vi "Main.vi"() -> ()   [LabVIEW 2012]
uses:
  UIActionQueueElement.ctl
  UIAction.ctl
  MemoryGlobalAction.ctl
  ScanListGlobalAction.ctl
  TriggerConfigurationGlobalAction.ctl
  SlotConfigurationGlobalAction.ctl
  Setup.ctl
  SlotConfiguration.ctl
  BankConfiguration.ctl
  TriggerConfiguration.ctl
  TriggerArmConfiguration.ctl
  driver/Public/Controls/ArmSource.ctl
  TriggerScanConfiguration.ctl
  driver/Public/Controls/ScanSource.ctl
  TriggerChannelConfiguration.ctl
  driver/Public/Controls/TriggerSource.ctl
  HardwareActionQueueElement.ctl
  HardwareAction.ctl
  libs/LV-Utilities/LV-Utilities.lvlib
  driver/Keithley-7001.lvlib
panel:
  in  "Tab Control":enum32{"Page 1"}(tab)
  out "Setup File":path
  in  "CONFIGURE SLOT 1":bool
  in  "CONFIGURE MEMORY":bool
  in  "CONFIGURE SCAN":bool
  in  "CONFIGURE TRIGGER":bool
  in  "Hardware START":bool
  out "Hardware Running?":bool
  in  "RESET":bool
  in  "SAVE":bool
  in  "OPEN":bool
  in  "DONE":bool
  # "RUN"
  # "SETUP"
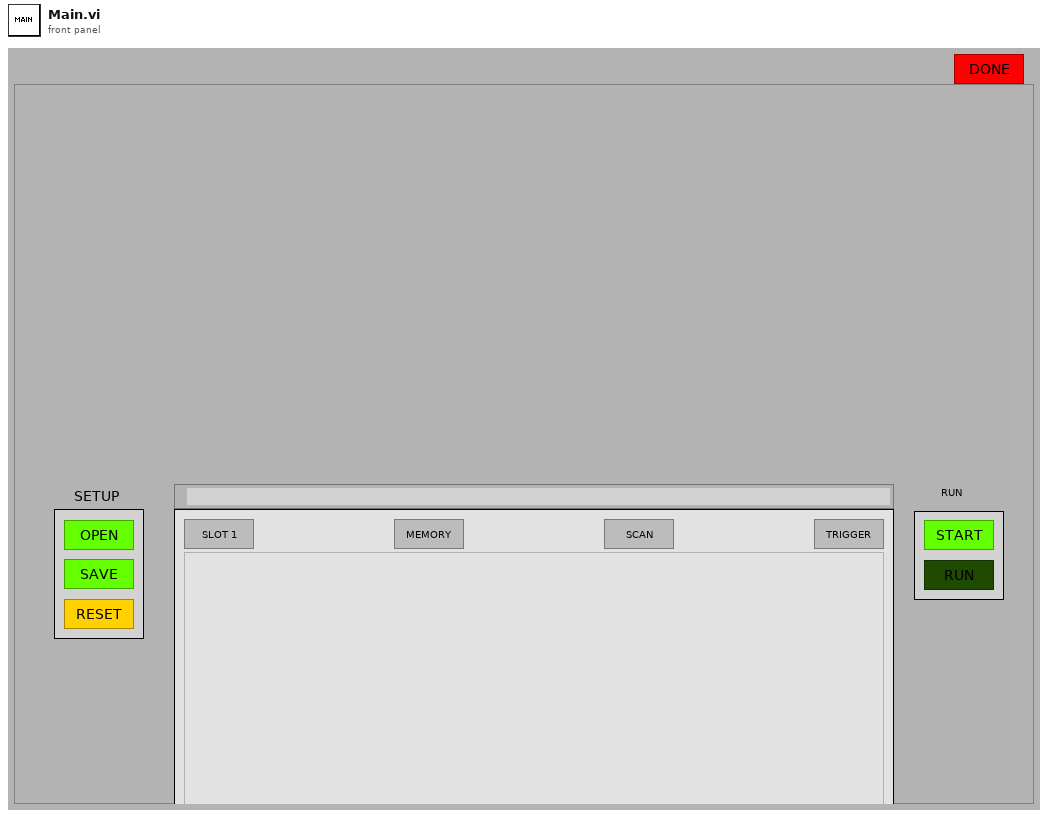
[diagram p1: front panel]
types:
  T1 = typedef "ActionQueues.ctl" = cluster{"User Interface":refnum<queue>, "Hardware":refnum<queue>}
  T2 = typedef "ExecutableConfiguration.ctl" = cluster{"GPIB ID":u8, "GPIB Board":u8, "Default Setup Folder":path}
  T3 = typedef "SlotConfigurationGlobalAction.ctl" = enum16{"Get", "Set", "Reset"}
  T4 = typedef "TriggerConfigurationGlobalAction.ctl" = enum16{"Get", "Set", "Reset"}
  T5 = typedef "ScanListGlobalAction.ctl" = enum16{"Get", "Set", "Reset"}
  T6 = typedef "MemoryGlobalAction.ctl" = enum16{"Get", "Set", "Reset"}
  T7 = typedef "Setup.ctl" = cluster{"Slots":T8[], "Memory":string[], "Scan List":string, "Trigger":T10}
  T8 = typedef "SlotConfiguration.ctl" = cluster{"Board":string, "Name":string, "Banks":T9[]}
  T9 = typedef "BankConfiguration.ctl" = cluster{"ID":string, "Name":string, "Channel Names":string[]}
  T10 = typedef "TriggerConfiguration.ctl" = cluster{"Arm":T11, "Scan":T13, "Channel":T15}
  T11 = typedef "TriggerArmConfiguration.ctl" = cluster{"Source":T12, "Count":u32, "Infinite?":bool}
  T12 = typedef "Keithley-7001.lvlib/ArmSource.ctl" = enum16{"Hold", "Immediate", "Manual", "Bus", "TLink", "External"}
  T13 = typedef "TriggerScanConfiguration.ctl" = cluster{"Source":T14, "Count":u32, "Infinite?":bool, "Delay (sec)":dbl, "Interval (sec)":dbl}
  T14 = typedef "Keithley-7001.lvlib/ScanSource.ctl" = enum16{"Hold", "Immediate", "Timer", "Manual", "Bus", "TLink", "External"}
  T15 = typedef "TriggerChannelConfiguration.ctl" = cluster{"Source":T16, "Count":u32, "Infinite?":bool, "Auto Count?":bool, "Delay (sec)":dbl, "Interval (sec)":dbl}
  T16 = typedef "Keithley-7001.lvlib/TriggerSource.ctl" = enum16{"Hold", "Immediate", "Manual", "Bus", "TLink", "External", "Timer"}
  T17 = typedef "HardwareActionQueueElement.ctl" = cluster{"Action":T18, "Data":variant}
  T18 = typedef "HardwareAction.ctl" = enum16{"Initialize", "Start", "Stop", "Error", "Shutdown"}
  T19 = typedef "UIActionQueueElement.ctl" = cluster{"Action":T20, "Data":variant}
  T20 = typedef "UIAction.ctl" = enum16{"Initialize", "Configure Trigger", "Configure Scan", "Configure Memory", "Configure Slot 1", "Open", "Save", "Reset", "Start", "Started", "Stop", "Stopped", "Shutdown"}
  T21 = enum8{"Enabled", "Disabled", "Disabled and Grayed Out"}
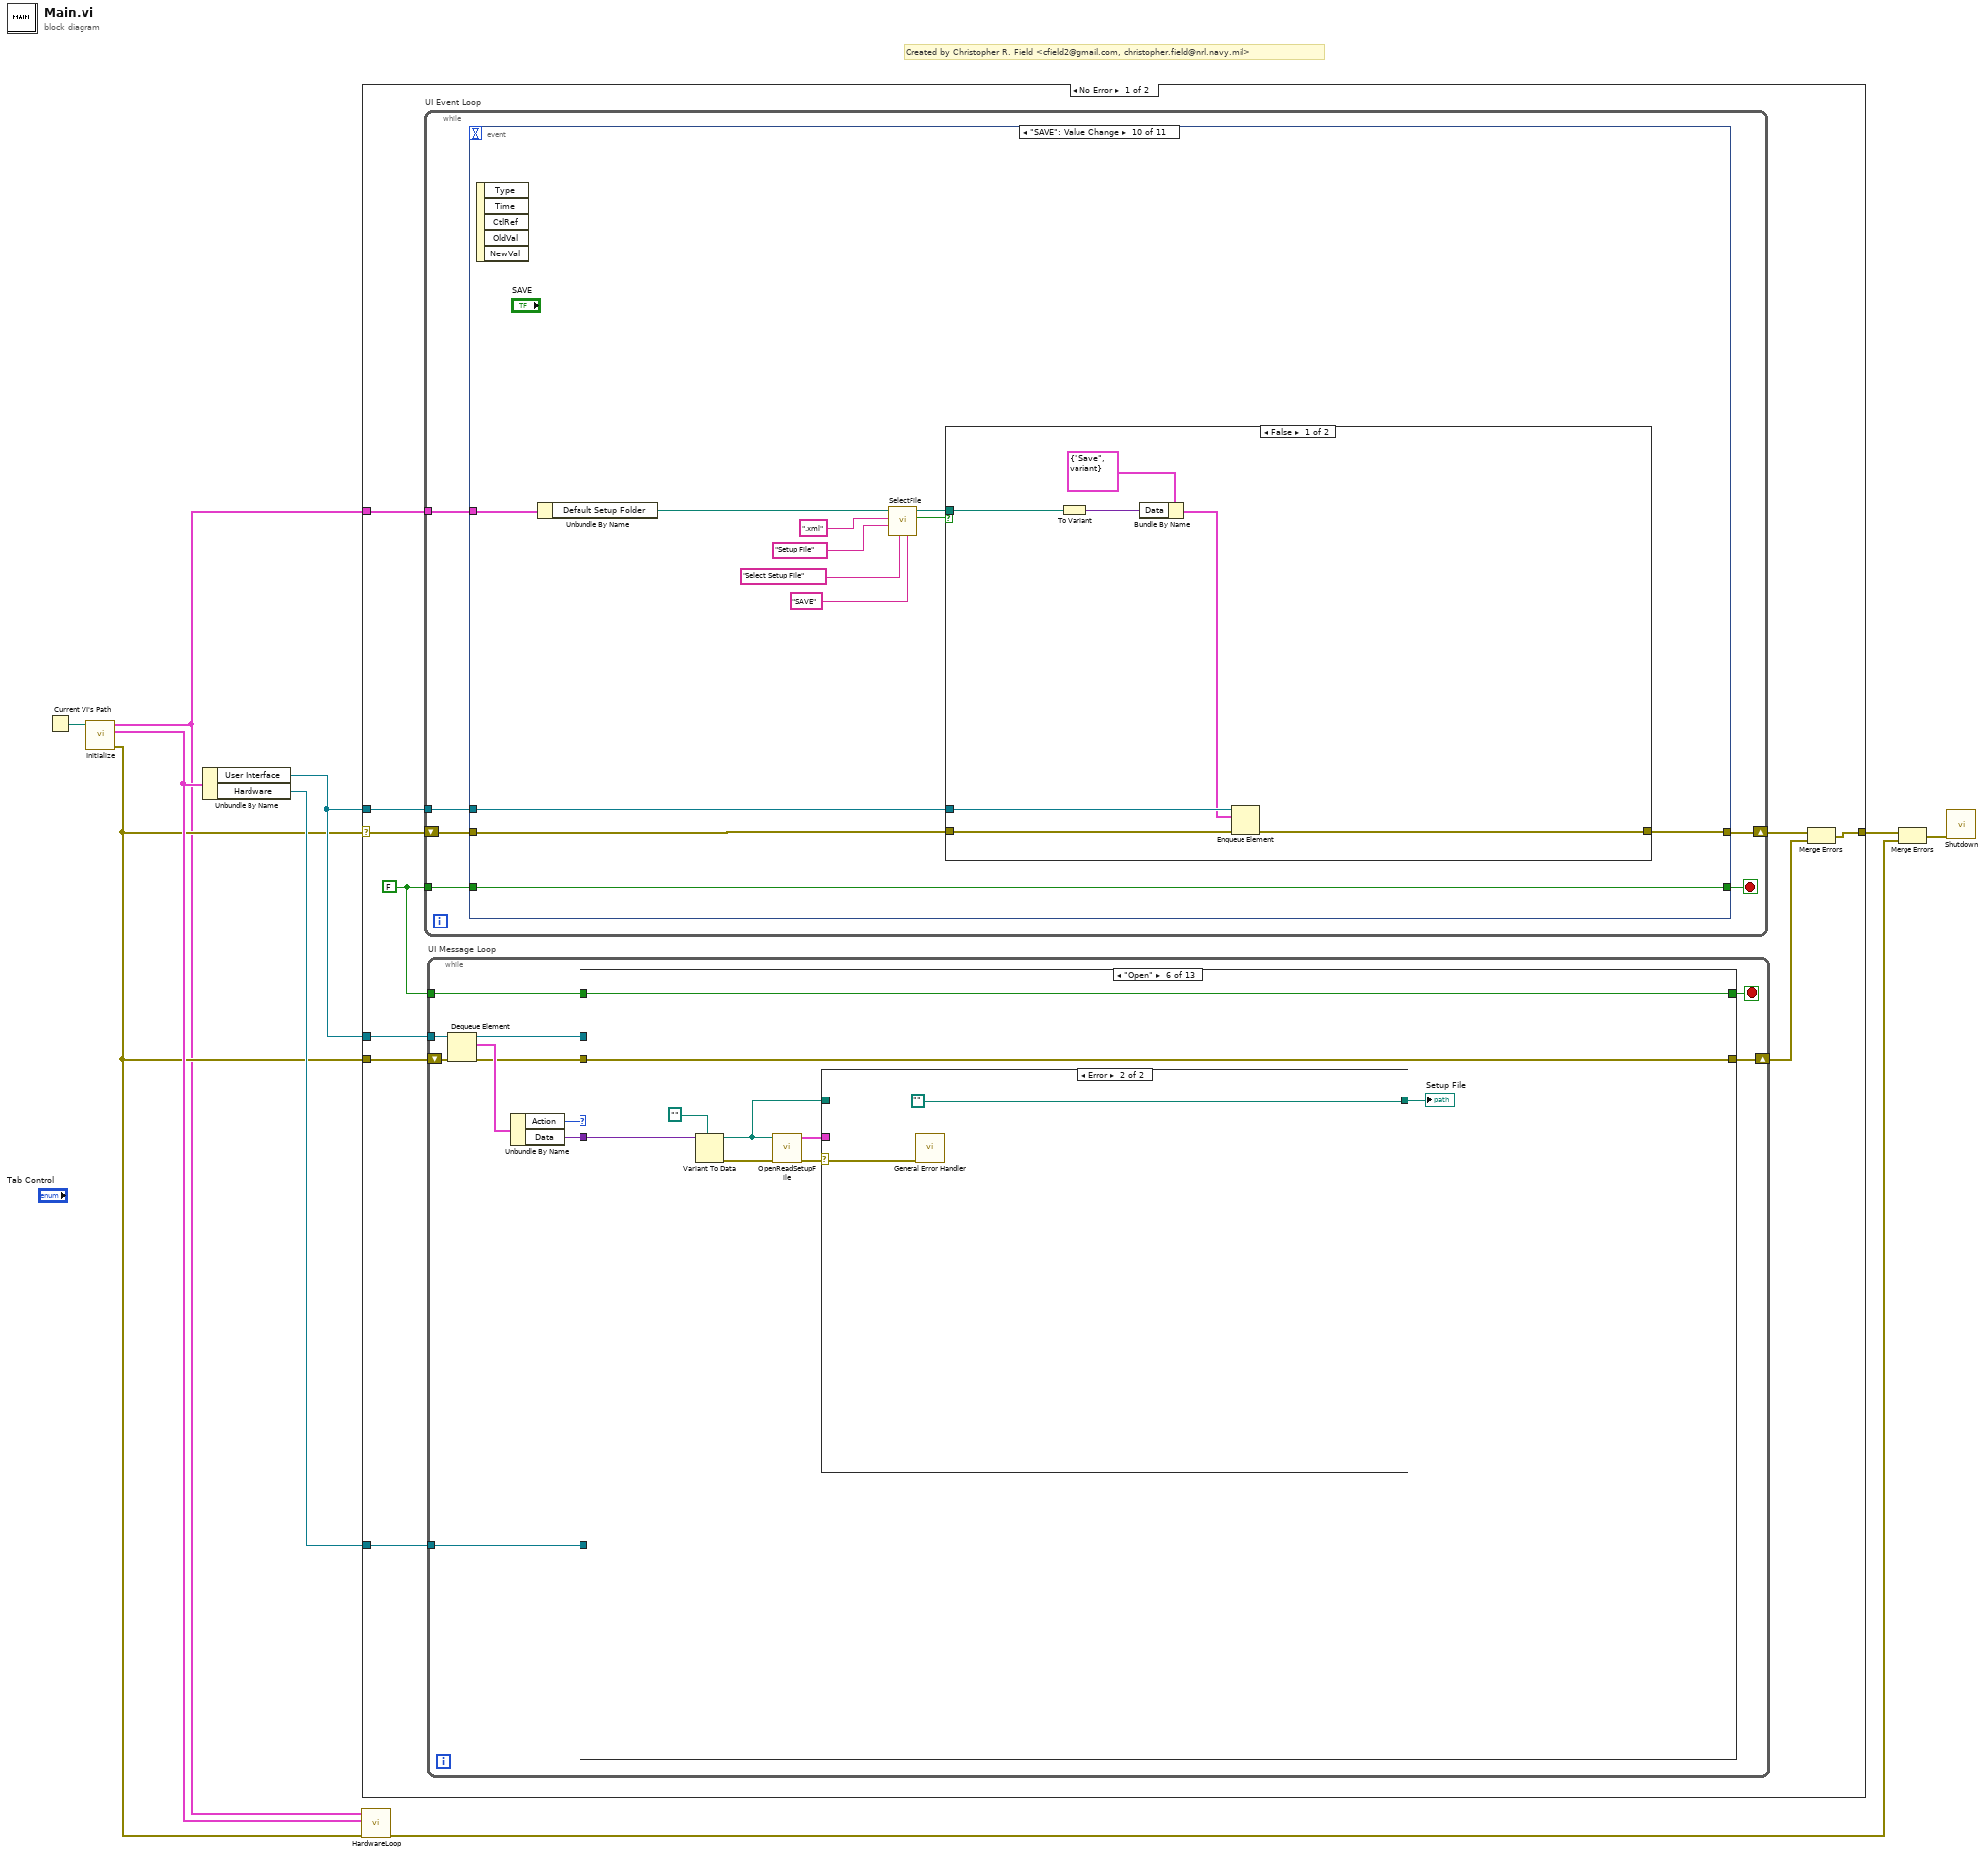
[diagram p0: block diagram]
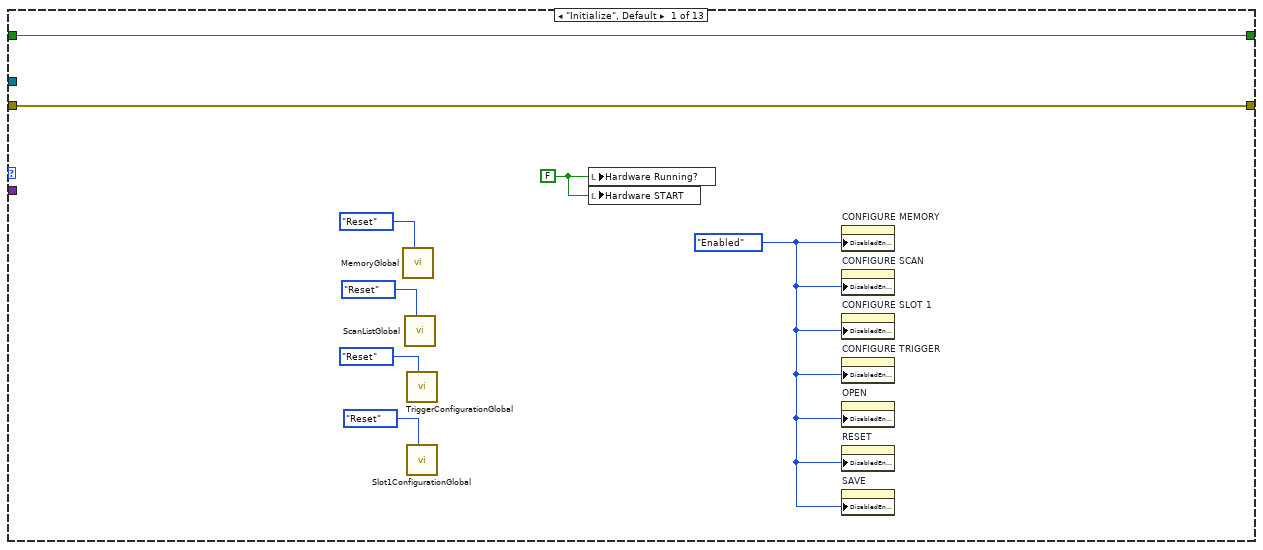
[diagram p2: hidden frame]
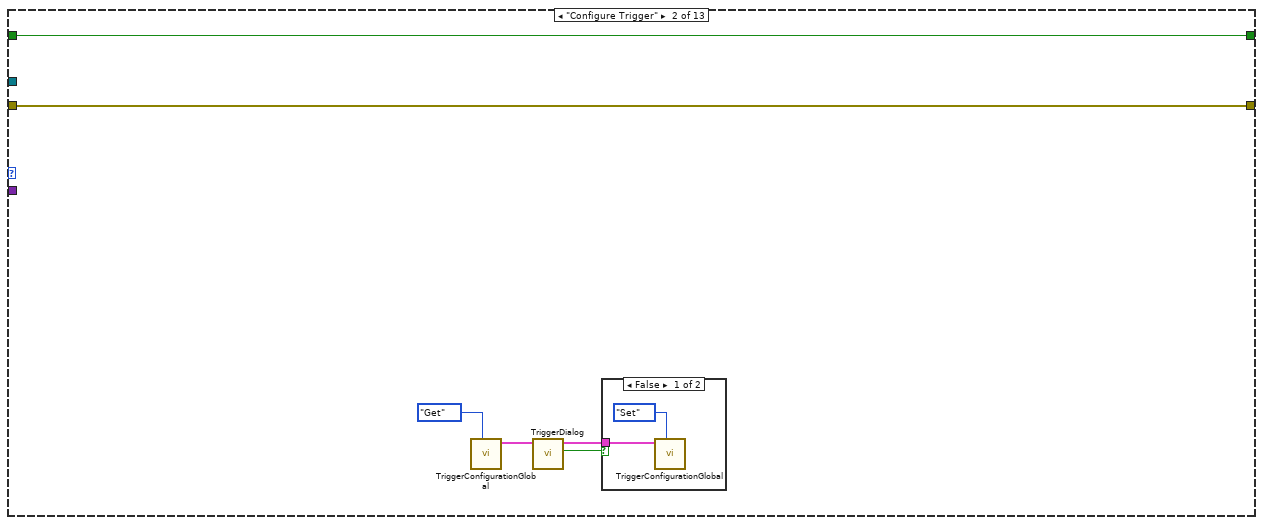
[diagram p3: hidden frame]
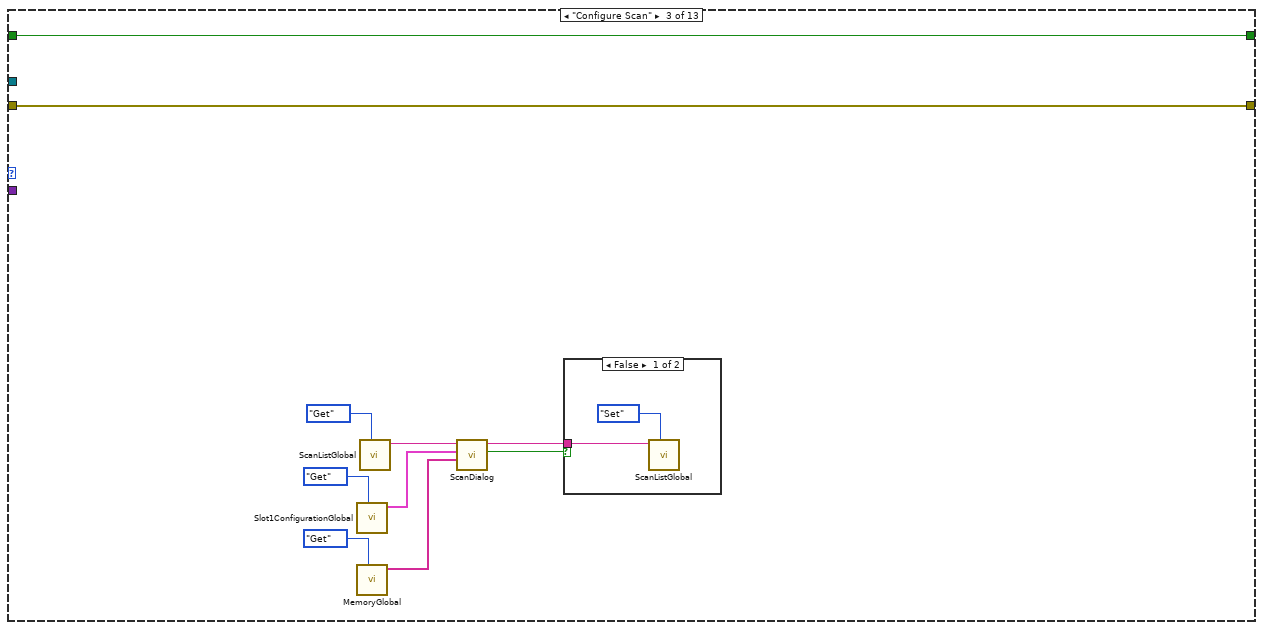
[diagram p5: hidden frame]
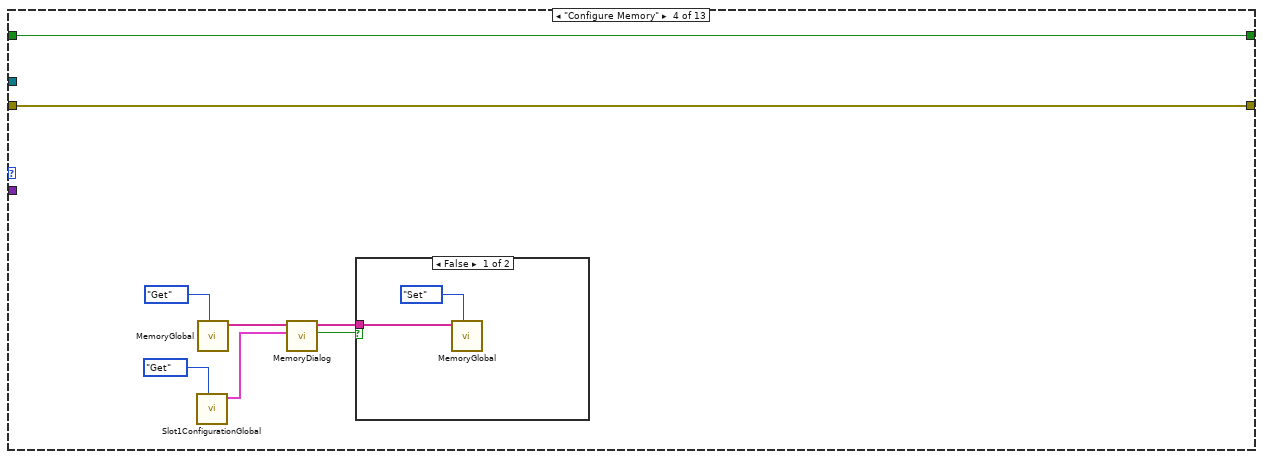
[diagram p7: hidden frame]
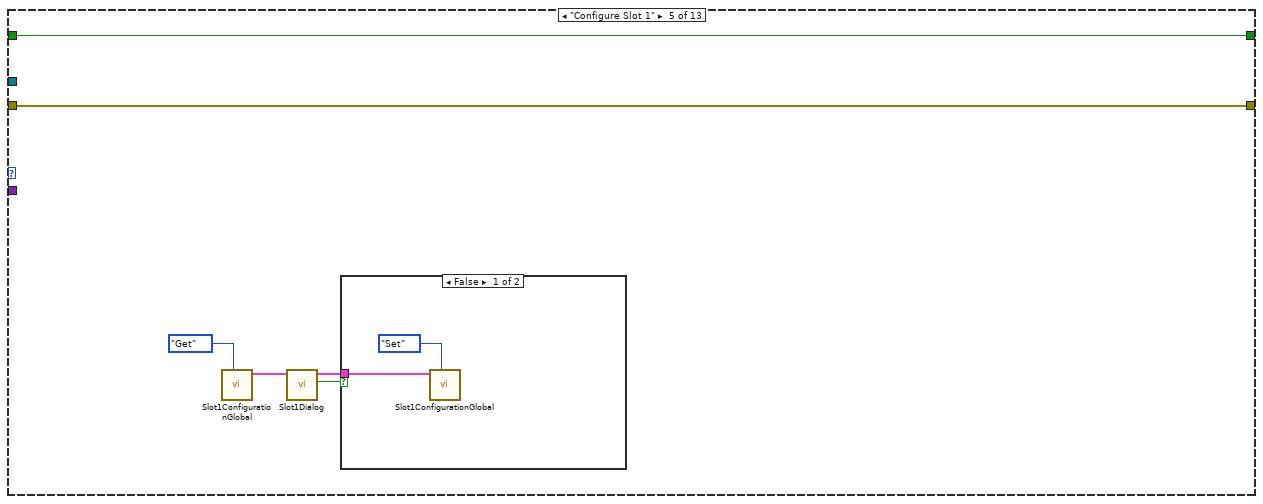
[diagram p9: hidden frame]
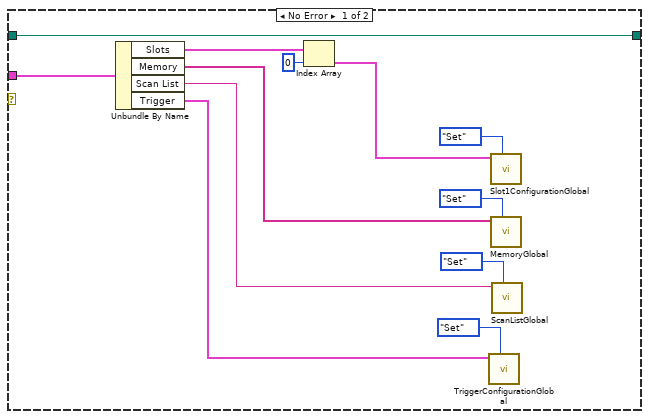
[diagram p11: hidden frame]
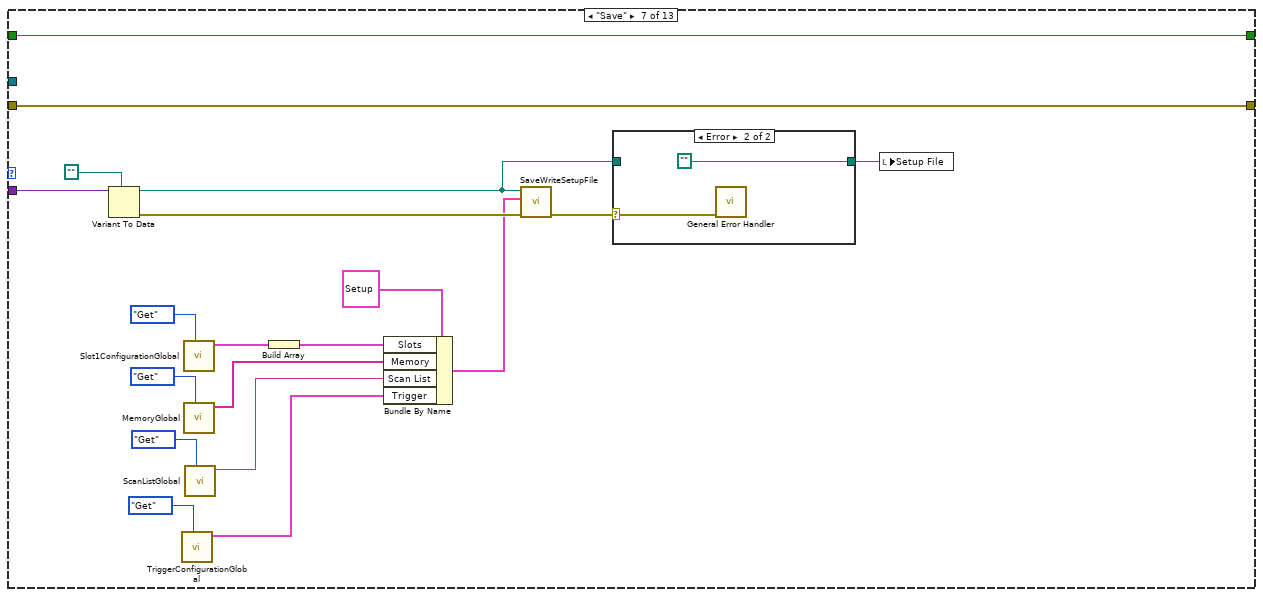
[diagram p12: hidden frame]
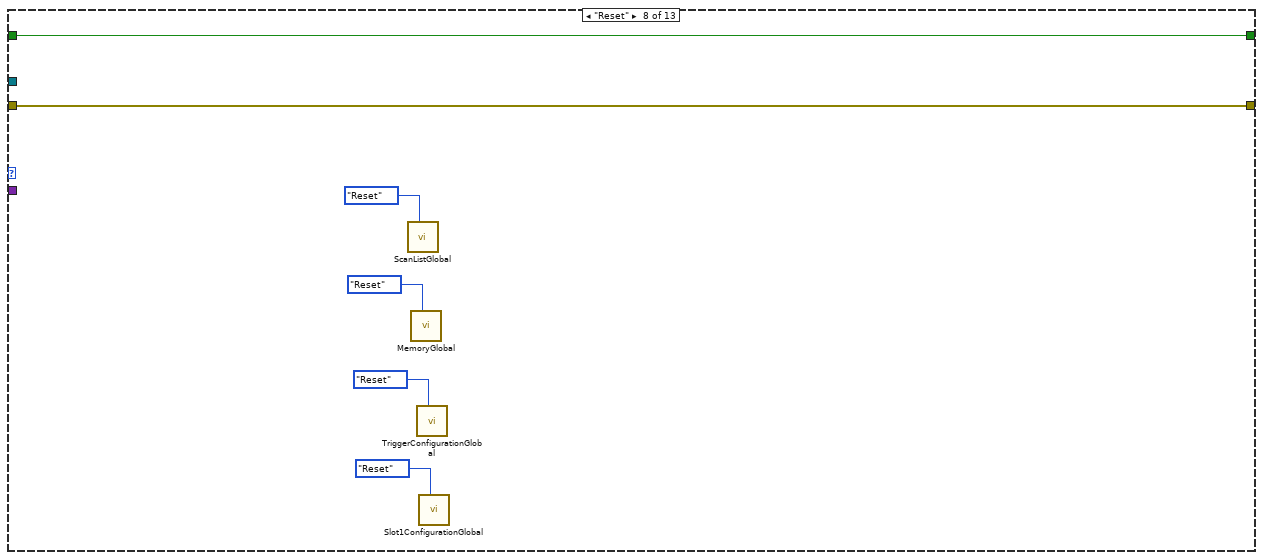
[diagram p14: hidden frame]
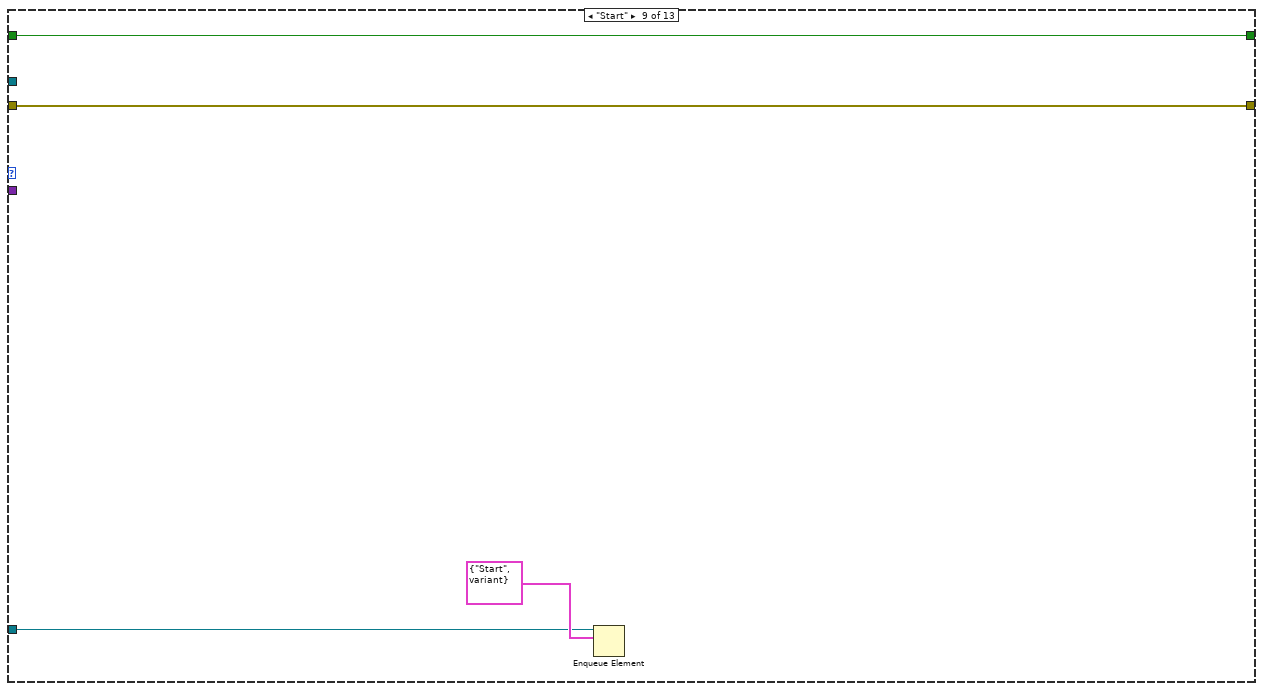
[diagram p15: hidden frame]
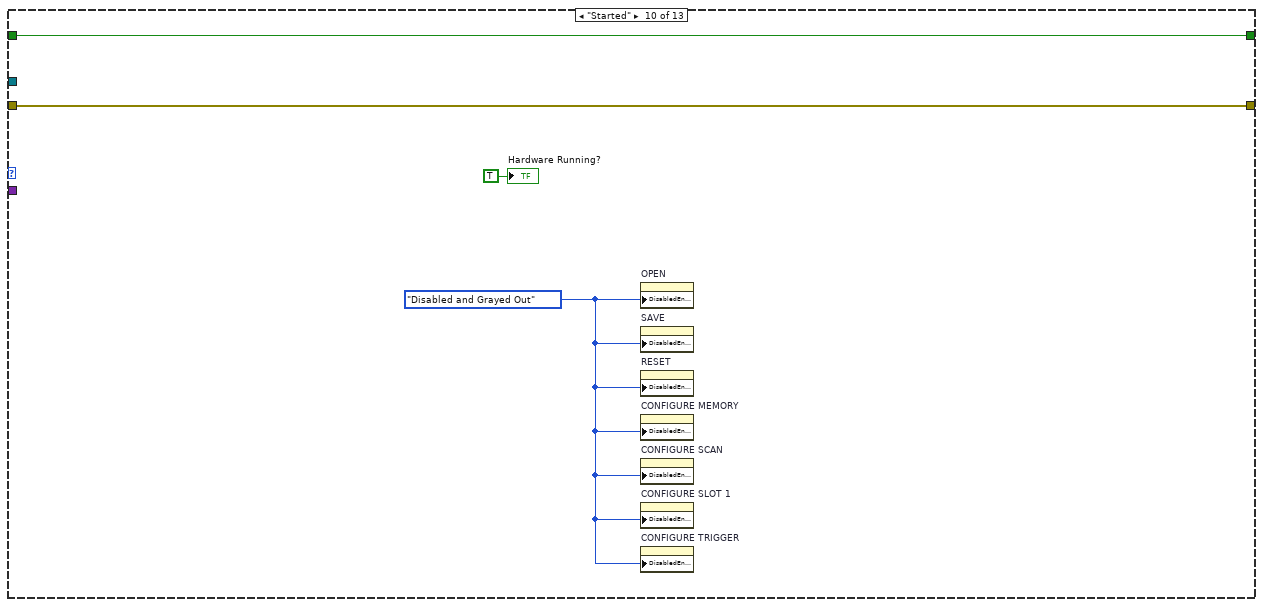
[diagram p16: hidden frame]
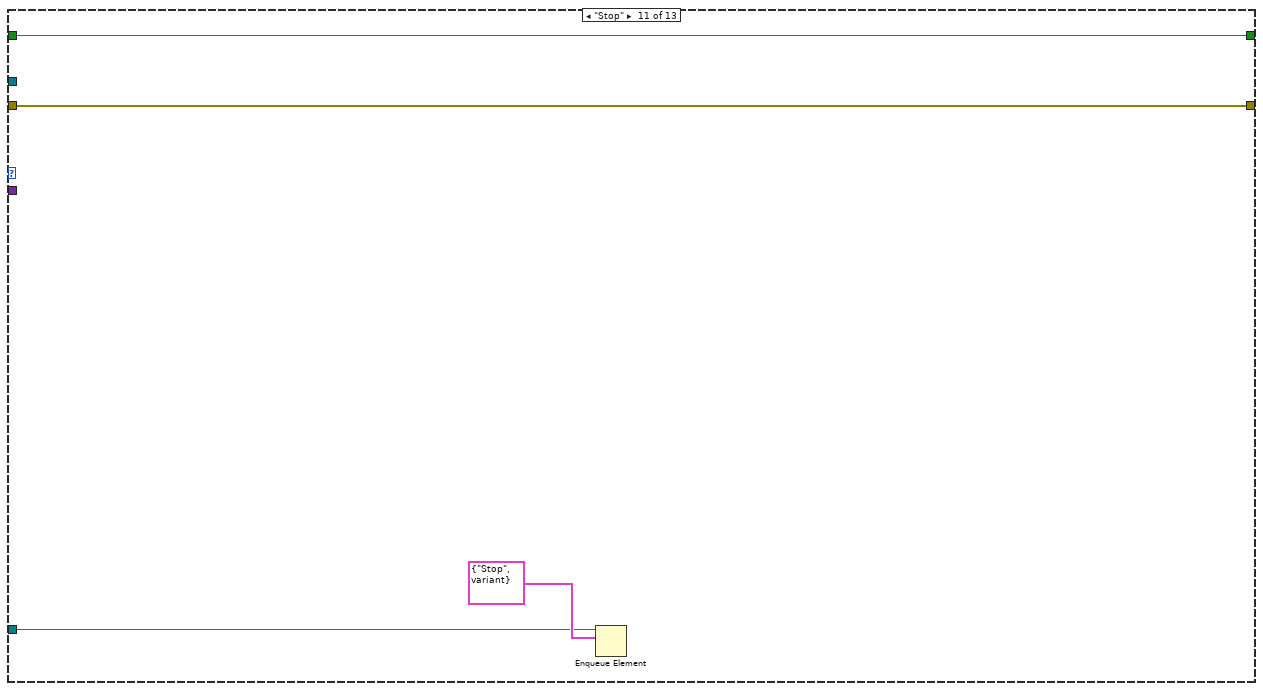
[diagram p17: hidden frame]
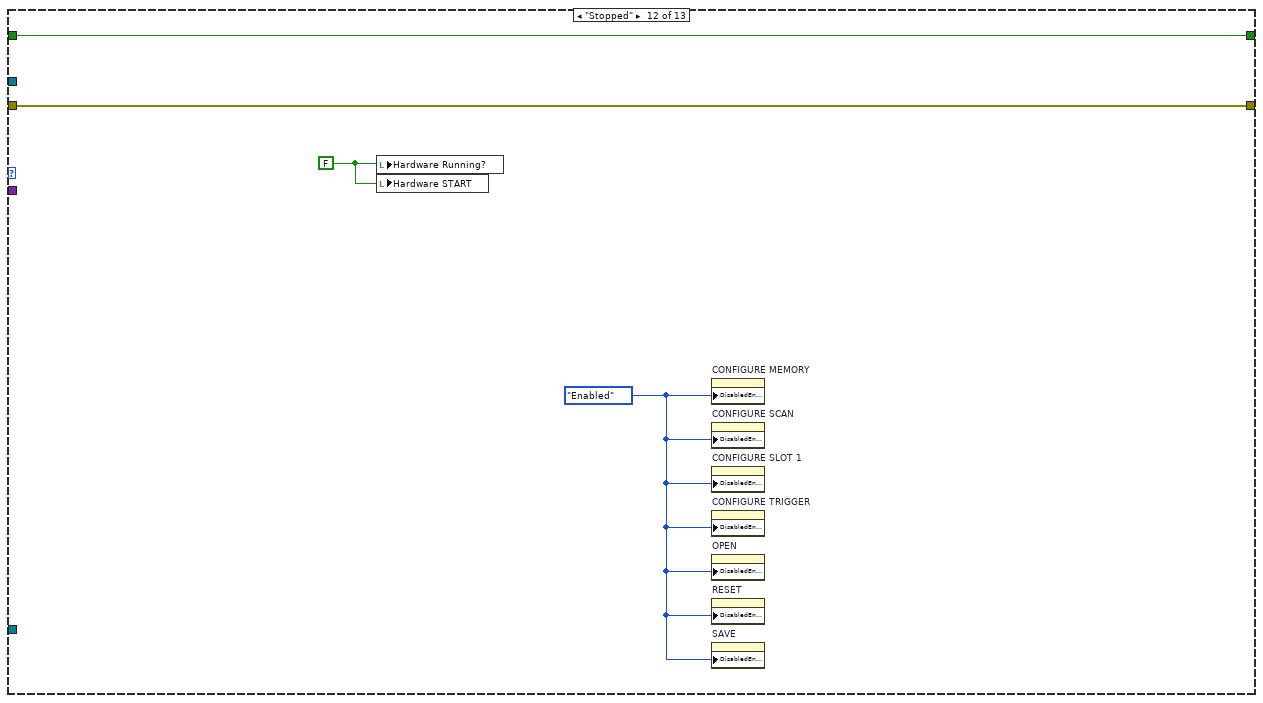
[diagram p18: hidden frame]
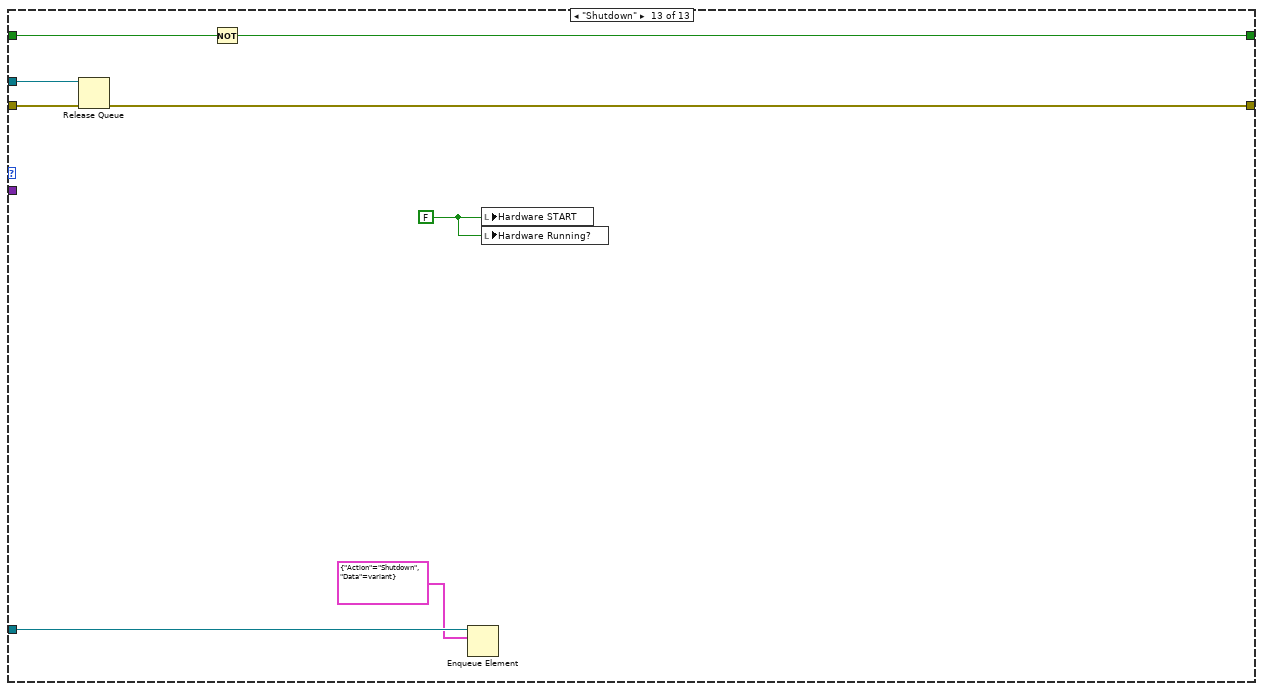
[diagram p19: hidden frame]
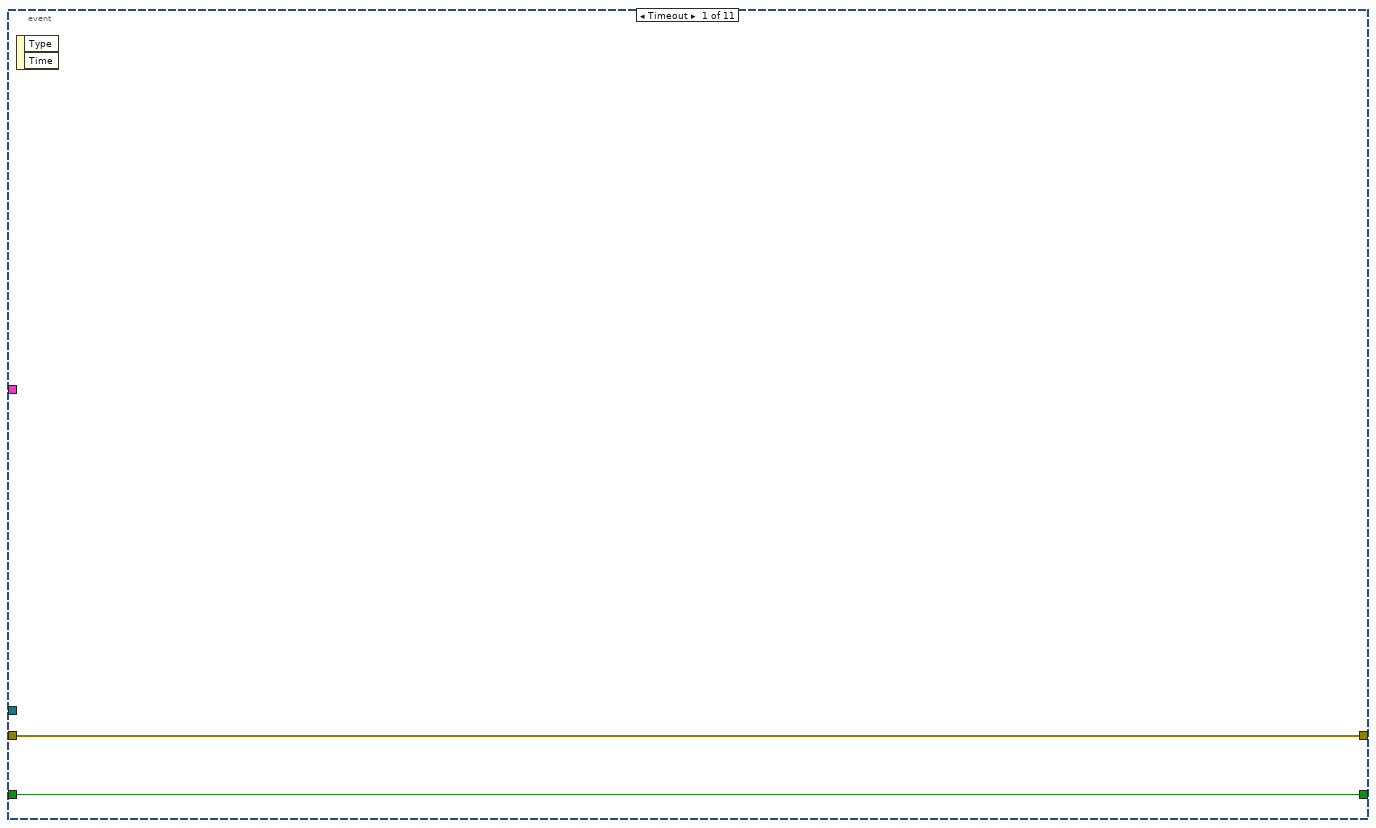
[diagram p20: hidden frame]
diagram:
  # "Created by Christopher R. Field <cfield2@gmail.com, christopher.field@nrl.navy.mil>"
  n1 = Current VI's Path() -> (path=w9:path)
  n2 = call "Initialize.vi"("VI Path"=w9) -> ("Error Out"=w5:errorcluster, "Action Queues"=w6:T1, "Executable Configuration"=w1:T2)  [unwired: 8 in]
  n3 = Unbundle By Name(w6) -> ("User Interface"=w8:refnum<queue>, "Hardware"=w7:refnum<queue>)
  n4 = call "HardwareLoop.vi"("Error In"=w5, "Action Queues"=w6, "Executable Configuration"=w1) -> ("Error Out"=w2:errorcluster)  [unwired: 8 in]
  n5 = case shown="No Error" w5 {
    selector: w5 -> [w19 w242]
    tunnel: [w12 w242] -> w4
    tunnel: w8 -> [w17 _]
    tunnel: w8 -> [w16 _]
    tunnel: w5 -> [w15 _]
    tunnel: w7 -> [w11 _]
    tunnel: w1 -> [w10 _]
    frame No Error {
      w18 = FALSE
      n6 = while "UI Event Loop" {
        shift-right: [w156] -> w14
        shift-left: w19 -> [w157]
        tunnel: w18 -> [w155]
        tunnel: w17 -> [w153]
        tunnel: w10 -> [w152]
        stop <- w154 stop-if-true
        n7 = event shown="[9] \"SAVE\": Value Change" {
          selector: _ -> [_ _ _ _ _ _ _ _ _ _ _]
          dyn-events: _ -> [_ _ _ _ _ _ _ _ _ _ _]
          timeout: _ -> [_ _ _ _ _ _ _ _ _ _ _]
          tunnel: w157 -> [w159 w162 w165 w172 w179 w185 w190 w194 w197 w219 w240]
          tunnel: [w159 w162 w164 w171 w175 w183 w189 w193 w198 w218 w239] -> w156
          tunnel: w155 -> [w158 w161 w168 w170 w174 w182 w188 w196 w202 w217 w238]
          tunnel: [w158 w160 w167 w170 w174 w182 w188 w196 w202 w217 w238] -> w154
          tunnel: w153 -> [_ _ w166 w173 w180 w186 w191 w195 w199 w220 w241]
          tunnel: w152 -> [_ _ _ _ _ _ _ _ w208 w221 _]
          event Timeout {
            n8 = event-data() -> ()  [unwired: 1 in, 2 out]
          }
          event Panel Close? {
            n9 = event-data() -> ()  [unwired: 1 in, 3 out]
            n10 = Not(x=w161) -> (.not. x?=w160:bool)
            n11 = event-data("Discard?"=w160) -> ()  [unwired: 1 in, 1 out]
          }
          event "DONE": Value Change {
            n12 = event-data() -> ()  [unwired: 1 in, 5 out]
            n13 = Not(x=w168) -> (.not. x?=w167:bool)
            n14 = Enqueue Element(queue=w166, element=T19 {"Action"=enum."Shutdown", "Data"=variant}, error in (no error)=w165) -> (error out=w164:errorcluster)  [unwired: 1 in, 2 out]
          }
          event "CONFIGURE TRIGGER": Value Change {
            n15 = event-data() -> ()  [unwired: 1 in, 5 out]
            n16 = Enqueue Element(queue=w173, element=T19 {"Action"=enum."Configure Trigger", "Data"=variant}, error in (no error)=w172) -> (error out=w171:errorcluster)  [unwired: 1 in, 2 out]
          }
          event "Hardware START": Value Change {
            n17 = event-data() -> ()  [unwired: 1 in, 5 out]
            n18 = Select(t=T19 {"Action"=enum."Start", "Data"=variant} ("element"), s="Hardware START", f=T19 {"Action"=enum."Stop", "Data"=variant} ("element")) -> (s? t:f=w176:T19)
            n19 = Enqueue Element(queue=w180, element=w176, error in (no error)=w179) -> (error out=w175:errorcluster)  [unwired: 1 in, 2 out]
          }
          event "CONFIGURE SCAN": Value Change {
            n20 = event-data() -> ()  [unwired: 1 in, 5 out]
            n21 = Enqueue Element(queue=w186, element=T19 {"Action"=enum."Configure Scan", "Data"=variant}, error in (no error)=w185) -> (error out=w183:errorcluster)  [unwired: 1 in, 2 out]
          }
          event "CONFIGURE MEMORY": Value Change {
            n22 = event-data() -> ()  [unwired: 1 in, 5 out]
            n23 = Enqueue Element(queue=w191, element=T19 {"Action"=enum."Configure Memory", "Data"=variant}, error in (no error)=w190) -> (error out=w189:errorcluster)  [unwired: 1 in, 2 out]
          }
          event "CONFIGURE SLOT 1": Value Change {
            n24 = event-data() -> ()  [unwired: 1 in, 5 out]
            n25 = Enqueue Element(queue=w195, element=T19 {"Action"=enum."Configure Slot 1", "Data"=variant}, error in (no error)=w194) -> (error out=w193:errorcluster)  [unwired: 1 in, 2 out]
          }
          event "OPEN": Value Change {
            n26 = event-data() -> ()  [unwired: 1 in, 5 out]
            n27 = Unbundle By Name(w208) -> ("Default Setup Folder"=w207:path)
            n28 = call "SelectFile.vi"("Button Label"="OPEN", "Prompt"="Select Setup File", "File Description"="Setup File", "File Extension (.*)"=".xml", "Start Path"=w207) -> ("Cancelled?"=w201:bool, "Selected File Path"=w200:path)  [unwired: 4 in, 1 out]
            n29 = case shown="False" w201 {
              tunnel: w200 -> [w210 _]
              tunnel: w199 -> [w215 _]
              tunnel: [w214 w216] -> w198
              tunnel: w197 -> [w213 w216]
              frame False {
                n30 = To Variant(anything=w210) -> (Variant=w211:variant)
                n31 = Bundle By Name(cluster=T19 {"Action"=enum."Open", "Data"=variant} ("element"), "Data"=w211) -> (w209:T19)
                n32 = Enqueue Element(queue=w215, element=w209, error in (no error)=w213) -> (error out=w214:errorcluster)  [unwired: 1 in, 2 out]
              }
              frame True {
              }
            }
          }
          event "SAVE": Value Change {
            n33 = event-data() -> ()  [unwired: 1 in, 5 out]
            n34 = Unbundle By Name(w221) -> ("Default Setup Folder"=w228:path)
            n35 = call "SelectFile.vi"("Button Label"="SAVE", "Prompt"="Select Setup File", "File Description"="Setup File", "File Extension (.*)"=".xml", "Start Path"=w228) -> ("Cancelled?"=w223:bool, "Selected File Path"=w222:path)  [unwired: 4 in, 1 out]
            n36 = case shown="False" w223 {
              tunnel: w222 -> [w230 _]
              tunnel: w220 -> [w235 _]
              tunnel: [w234 w236] -> w218
              tunnel: w219 -> [w233 w236]
              frame False {
                n37 = To Variant(anything=w230) -> (Variant=w231:variant)
                n38 = Bundle By Name(cluster=T19 {"Action"=enum."Save", "Data"=variant} ("element"), "Data"=w231) -> (w229:T19)
                n39 = Enqueue Element(queue=w235, element=w229, error in (no error)=w233) -> (error out=w234:errorcluster)  [unwired: 1 in, 2 out]
              }
              frame True {
              }
            }
          }
          event "RESET": Value Change {
            n40 = event-data() -> ()  [unwired: 1 in, 5 out]
            n41 = Enqueue Element(queue=w241, element=T19 {"Action"=enum."Reset", "Data"=variant}, error in (no error)=w240) -> (error out=w239:errorcluster)  [unwired: 1 in, 2 out]
          }
        }
      }
      n42 = while "UI Message Loop" {
        tunnel: w18 -> [w30]
        tunnel: w16 -> [w29]
        shift-right: [w22] -> w13
        shift-left: w15 -> [w28]
        tunnel: w11 -> [w20]
        stop <- w21 stop-if-true
        n43 = Dequeue Element(queue=w29, error in (no error)=w28) -> (queue out=w23:refnum<queue>, element=w27:T19, error out=w24:errorcluster)  [unwired: 1 in, 1 out]
        n44 = Unbundle By Name(w27) -> ("Action"=w26:T20, "Data"=w25:variant)
        n45 = case shown="\"Open\"" w26 {
          tunnel: w30 -> [w38 w43 w56 w66 w73 w85 w117 w127 w131 w135 w139 w143 w151]
          tunnel: w25 -> [_ _ _ _ _ w83 w116 _ _ _ _ _ _]
          tunnel: w24 -> [w37 w44 w55 w65 w74 w84 w118 w126 w130 w134 w138 w142 w148]
          tunnel: w23 -> [_ _ _ _ _ _ _ _ _ _ _ _ w149]
          tunnel: [w37 w44 w55 w65 w74 w84 w118 w126 w130 w134 w138 w142 w147] -> w22
          tunnel: [w38 w43 w56 w66 w73 w85 w117 w127 w131 w135 w139 w143 w150] -> w21
          tunnel: w20 -> [_ _ _ _ _ _ _ _ w128 _ w136 _ w146]
          frame "Initialize", Default {
            w31 = T21."Enabled" ("Disabled")
            w36 = FALSE ("Hardware Running?")
            n46 = call "MemoryGlobal.vi"("Action"=MemoryGlobalAction."Reset") -> ()  [unwired: 10 in, 1 out]
            n47 = call "ScanListGlobal.vi"("Action"=ScanListGlobalAction."Reset") -> ()  [unwired: 10 in, 1 out]
            n48 = call "TriggerConfigurationGlobal.vi"("Action"=TriggerConfigurationGlobalAction."Reset") -> ()  [unwired: 10 in, 1 out]
            n49 = call "Slot1ConfigurationGlobal.vi"("Action"=SlotConfigurationGlobalAction."Reset") -> ()  [unwired: 10 in, 1 out]
            n50 = local write "Hardware Running?"(w36) -> ()
            n51 = local write "Hardware START"(w36) -> ()
            n52 = property on="CONFIGURE MEMORY" class="Bool"("DisabledEnum"=w31) -> ()  [unwired: 2 in, 2 out]
            n53 = property on="CONFIGURE SCAN" class="Bool"("DisabledEnum"=w31) -> ()  [unwired: 2 in, 2 out]
            n54 = property on="CONFIGURE SLOT 1" class="Bool"("DisabledEnum"=w31) -> ()  [unwired: 2 in, 2 out]
            n55 = property on="CONFIGURE TRIGGER" class="Bool"("DisabledEnum"=w31) -> ()  [unwired: 2 in, 2 out]
            n56 = property on="OPEN" class="Bool"("DisabledEnum"=w31) -> ()  [unwired: 2 in, 2 out]
            n57 = property on="RESET" class="Bool"("DisabledEnum"=w31) -> ()  [unwired: 2 in, 2 out]
            n58 = property on="SAVE" class="Bool"("DisabledEnum"=w31) -> ()  [unwired: 2 in, 2 out]
          }
          frame "Configure Trigger" {
            n59 = call "TriggerConfigurationGlobal.vi"("Action"=TriggerConfigurationGlobalAction."Get") -> ("Value Out"=w41:T10)  [unwired: 10 in]
            n60 = call "TriggerDialog.vi"("Trigger Configuration In"=w41) -> ("Cancelled?"=w39:bool, "Trigger Configuration Out"=w40:T10)  [unwired: 8 in, 1 out]
            n61 = case shown="False" w39 {
              tunnel: w40 -> [w46 _]
              frame False {
                n62 = call "TriggerConfigurationGlobal.vi"("Action"=TriggerConfigurationGlobalAction."Set", "Set Value"=w46) -> ()  [unwired: 9 in, 1 out]
              }
              frame True {
              }
            }
          }
          frame "Configure Scan" {
            n63 = call "Slot1ConfigurationGlobal.vi"("Action"=SlotConfigurationGlobalAction."Get") -> ("Value Out"=w49:T8)  [unwired: 10 in]
            n64 = call "MemoryGlobal.vi"("Action"=MemoryGlobalAction."Get") -> ("Value Out"=w47:string[])  [unwired: 10 in]
            n65 = call "ScanListGlobal.vi"("Action"=ScanListGlobalAction."Get") -> ("Value Out"=w53:string)  [unwired: 10 in]
            n66 = call "ScanDialog.vi"("Channel Patterns"=w47, "Slot Configuration"=w49, "Scan List In"=w53) -> ("Cancelled?"=w51:bool, "Scan List Out"=w52:string)  [unwired: 6 in, 1 out]
            n67 = case shown="False" w51 {
              tunnel: w52 -> [w57 _]
              frame False {
                n68 = call "ScanListGlobal.vi"("Action"=ScanListGlobalAction."Set", "Set Value"=w57) -> ()  [unwired: 9 in, 1 out]
              }
              frame True {
              }
            }
          }
          frame "Configure Memory" {
            n69 = call "Slot1ConfigurationGlobal.vi"("Action"=SlotConfigurationGlobalAction."Get") -> ("Value Out"=w59:T8)  [unwired: 10 in]
            n70 = call "MemoryGlobal.vi"("Action"=MemoryGlobalAction."Get") -> ("Value Out"=w63:string[])  [unwired: 10 in]
            n71 = call "MemoryDialog.vi"("Slot 1 Configuration"=w59, "Channel Patterns In"=w63) -> ("Cancelled?"=w62:bool, "Channel Patterns Out"=w61:string[])  [unwired: 7 in, 1 out]
            n72 = case shown="False" w62 {
              tunnel: w61 -> [w68 _]
              frame False {
                n73 = call "MemoryGlobal.vi"("Action"=MemoryGlobalAction."Set", "Set Value"=w68) -> ()  [unwired: 9 in, 1 out]
              }
              frame True {
              }
            }
          }
          frame "Configure Slot 1" {
            n74 = call "Slot1ConfigurationGlobal.vi"("Action"=SlotConfigurationGlobalAction."Get") -> ("Value Out"=w71:T8)  [unwired: 10 in]
            n75 = call "Slot1Dialog.vi"("Slot 1 Configuration In"=w71) -> ("Cancelled?"=w70:bool, "Slot 1 Configuration Out"=w69:T8)  [unwired: 8 in, 1 out]
            n76 = case shown="False" w70 {
              tunnel: w69 -> [w76 _]
              frame False {
                n77 = call "Slot1ConfigurationGlobal.vi"("Action"=SlotConfigurationGlobalAction."Set", "Set Value"=w76) -> ()  [unwired: 9 in, 1 out]
              }
              frame True {
              }
            }
          }
          frame "Open" {
            n78 = Variant To Data(type=path "", Variant=w83) -> (data=w80:path, error out=w81:errorcluster)  [unwired: 1 in]
            n79 = call "OpenReadSetupFile.vi"("Error In"=w81, "Setup File"=w80) -> ("Error Out"=w79:errorcluster, "Setup"=w78:T7)  [unwired: 8 in]
            n80 = case shown="Error" w79 {
              selector: w79 -> [_ w99]
              tunnel: w80 -> [w86 _]
              tunnel: w78 -> [w97 _]
              tunnel: [w86 path ""] -> w77
              frame No Error {
                n81 = Unbundle By Name(w97) -> ("Slots"=w92:T8[], "Memory"=w89:string[], "Scan List"=w88:string, "Trigger"=w87:T10)
                n82 = Index Array(array=w92, index=0) -> (element=w90:T8)
                n83 = call "TriggerConfigurationGlobal.vi"("Action"=TriggerConfigurationGlobalAction."Set", "Set Value"=w87) -> ()  [unwired: 9 in, 1 out]
                n84 = call "Slot1ConfigurationGlobal.vi"("Action"=SlotConfigurationGlobalAction."Set", "Set Value"=w90) -> ()  [unwired: 9 in, 1 out]
                n85 = call "MemoryGlobal.vi"("Action"=MemoryGlobalAction."Set", "Set Value"=w89) -> ()  [unwired: 9 in, 1 out]
                n86 = call "ScanListGlobal.vi"("Action"=ScanListGlobalAction."Set", "Set Value"=w88) -> ()  [unwired: 9 in, 1 out]
              }
              frame Error {
                n87 = call <vilib>:"General Error Handler.vi"("error in (no error)"=w99) -> ()  [unwired: 10 in, 5 out]
              }
            }
            "Setup File" <- w77
          }
          frame "Save" {
            n88 = Variant To Data(type=path "", Variant=w116) -> (data=w101:path, error out=w114:errorcluster)  [unwired: 1 in]
            n89 = call "TriggerConfigurationGlobal.vi"("Action"=TriggerConfigurationGlobalAction."Get") -> ("Value Out"=w105:T10)  [unwired: 10 in]
            n90 = call "Slot1ConfigurationGlobal.vi"("Action"=SlotConfigurationGlobalAction."Get") -> ("Value Out"=w104:T8)  [unwired: 10 in]
            n91 = call "MemoryGlobal.vi"("Action"=MemoryGlobalAction."Get") -> ("Value Out"=w109:string[])  [unwired: 10 in]
            n92 = call "ScanListGlobal.vi"("Action"=ScanListGlobalAction."Get") -> ("Value Out"=w106:string)  [unwired: 10 in]
            n93 = Build Array(w104) -> (w103:T8[])
            n94 = Bundle By Name(cluster=T7 {"Slots"=[], "Memory"=[], "Scan List"="", "Trigger"={"Arm"={"Source"=enum."Hold", "Count"=0, "Infinite?"=FALSE}, "Scan"={"Source"=enum."Hold", "Count"=0, "Infinite?"=FALSE, "Delay (sec)"=0.0, "Interval (sec)"=0.0}, "Channel"={"Source"=enum."Hold", "Count"=0, "Infinite?"=FALSE, "Auto Count?"=FALSE, "Delay (sec)"=0.0, "Interval (sec)"=0.0}}} ("Setup"), "Slots"=w103, "Memory"=w109, "Scan List"=w106, "Trigger"=w105) -> (w111:T7)
            n95 = call "SaveWriteSetupFile.vi"("Error In"=w114, "Setup"=w111, "Save File"=w101) -> ("Error Out"=w102:errorcluster)  [unwired: 8 in]
            n96 = case shown="Error" w102 {
              selector: w102 -> [_ w120]
              tunnel: w101 -> [w119 _]
              tunnel: [w119 path ""] -> w100
              frame No Error {
              }
              frame Error {
                n97 = call <vilib>:"General Error Handler.vi"("error in (no error)"=w120) -> ()  [unwired: 10 in, 5 out]
              }
            }
            n98 = local write "Setup File"(w100) -> ()
          }
          frame "Reset" {
            n99 = call "ScanListGlobal.vi"("Action"=ScanListGlobalAction."Reset") -> ()  [unwired: 10 in, 1 out]
            n100 = call "MemoryGlobal.vi"("Action"=MemoryGlobalAction."Reset") -> ()  [unwired: 10 in, 1 out]
            n101 = call "TriggerConfigurationGlobal.vi"("Action"=TriggerConfigurationGlobalAction."Reset") -> ()  [unwired: 10 in, 1 out]
            n102 = call "Slot1ConfigurationGlobal.vi"("Action"=SlotConfigurationGlobalAction."Reset") -> ()  [unwired: 10 in, 1 out]
          }
          frame "Start" {
            n103 = Enqueue Element(queue=w128, element=T17 {"Action"=enum."Start", "Data"=variant}) -> ()  [unwired: 2 in, 3 out]
          }
          frame "Started" {
            w132 = T21."Disabled and Grayed Out" ("Disabled")
            n104 = property on="OPEN" class="Bool"("DisabledEnum"=w132) -> ()  [unwired: 2 in, 2 out]
            n105 = property on="SAVE" class="Bool"("DisabledEnum"=w132) -> ()  [unwired: 2 in, 2 out]
            n106 = property on="RESET" class="Bool"("DisabledEnum"=w132) -> ()  [unwired: 2 in, 2 out]
            n107 = property on="CONFIGURE MEMORY" class="Bool"("DisabledEnum"=w132) -> ()  [unwired: 2 in, 2 out]
            n108 = property on="CONFIGURE SCAN" class="Bool"("DisabledEnum"=w132) -> ()  [unwired: 2 in, 2 out]
            n109 = property on="CONFIGURE SLOT 1" class="Bool"("DisabledEnum"=w132) -> ()  [unwired: 2 in, 2 out]
            n110 = property on="CONFIGURE TRIGGER" class="Bool"("DisabledEnum"=w132) -> ()  [unwired: 2 in, 2 out]
            "Hardware Running?" <- TRUE ("Hardware Running?")
          }
          frame "Stop" {
            n111 = Enqueue Element(queue=w136, element=T17 {"Action"=enum."Stop", "Data"=variant}) -> ()  [unwired: 2 in, 3 out]
          }
          frame "Stopped" {
            w140 = T21."Enabled" ("Disabled")
            w141 = FALSE ("Hardware Running?")
            n112 = local write "Hardware Running?"(w141) -> ()
            n113 = local write "Hardware START"(w141) -> ()
            n114 = property on="CONFIGURE MEMORY" class="Bool"("DisabledEnum"=w140) -> ()  [unwired: 2 in, 2 out]
            n115 = property on="CONFIGURE SCAN" class="Bool"("DisabledEnum"=w140) -> ()  [unwired: 2 in, 2 out]
            n116 = property on="CONFIGURE SLOT 1" class="Bool"("DisabledEnum"=w140) -> ()  [unwired: 2 in, 2 out]
            n117 = property on="CONFIGURE TRIGGER" class="Bool"("DisabledEnum"=w140) -> ()  [unwired: 2 in, 2 out]
            n118 = property on="OPEN" class="Bool"("DisabledEnum"=w140) -> ()  [unwired: 2 in, 2 out]
            n119 = property on="RESET" class="Bool"("DisabledEnum"=w140) -> ()  [unwired: 2 in, 2 out]
            n120 = property on="SAVE" class="Bool"("DisabledEnum"=w140) -> ()  [unwired: 2 in, 2 out]
          }
          frame "Shutdown" {
            w144 = FALSE ("Hardware START")
            n121 = Release Queue(queue=w149, error in (no error)=w148) -> (error out=w147:errorcluster)  [unwired: 1 in, 2 out]
            n122 = Not(x=w151) -> (.not. x?=w150:bool)
            n123 = Enqueue Element(queue=w146, element=T17 {"Action"=enum."Shutdown", "Data"=variant}) -> ()  [unwired: 2 in, 3 out]
            n124 = local write "Hardware START"(w144) -> ()
            n125 = local write "Hardware Running?"(w144) -> ()
          }
        }
      }
      n126 = Merge Errors(w14, w13) -> (w12:errorcluster)
    }
    frame Error {
    }
  }
  n127 = Merge Errors(w4, w2) -> (w3:errorcluster)
  n128 = call "Shutdown.vi"("Error In"=w3) -> ()  [unwired: 10 in, 1 out]
